vi "TEST_cRIO.vi"() -> ()   [LabVIEW 2017]
uses:
  <vilib>/Analysis/baseanly.llb/Mean (DBL).vi
  <vilib>/Analysis/NI_AALBase.lvlib
panel:
  in  "Boolean":bool
  out "R3(kOhm)":dbl format="%.1f"
  out "R2(kOhm)":dbl format="%.1f"
  out "R1(kOhm)":dbl format="%.1f"
  out "Corriente(mA)":dbl format="%.3f"
  in  "AO0":dbl format="%.2f"
  out "AI3(V)":dbl format="%.6f"
  out "AI2(V)":dbl format="%.6f"
  out "AI1(V)":dbl format="%.6f"
  out "Waveform Chart":cluster{dbl, dbl, dbl}(graph)
  in  "Period":dbl=0.1 format="%.1f"
  in  "stop":bool
  out "AI0(V)":dbl format="%.6f"
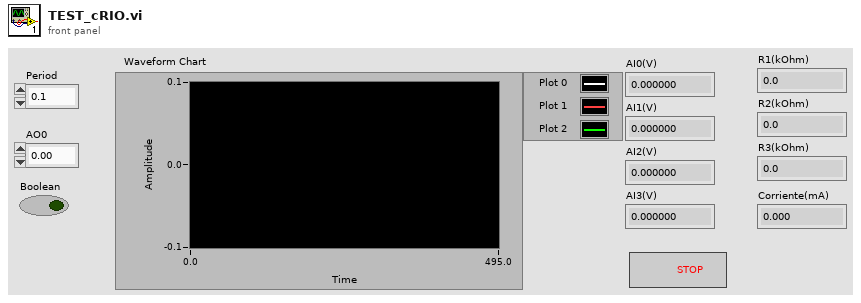
[diagram p1: front panel]
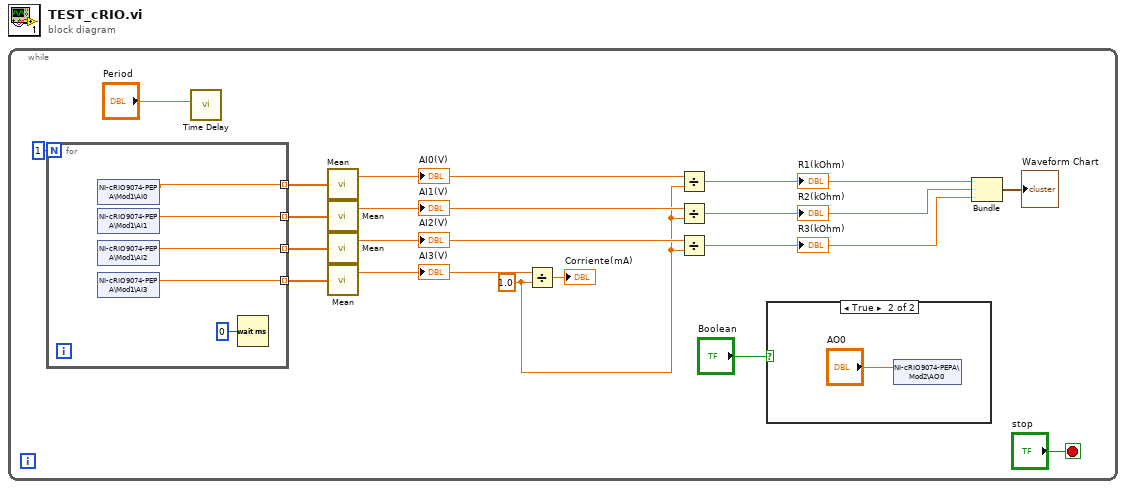
[diagram p0: block diagram]
diagram:
  n1 = while {
    stop <- "stop" stop-if-true
    w3 = 1.0 ("y")
    n2 = for {
      N: 1 -> [_]
      tunnel: [w20] -> w14 mode=indexing
      tunnel: [w21] -> w12 mode=indexing
      tunnel: [w22] -> w11 mode=indexing
      tunnel: [w23] -> w10 mode=indexing
      n3 = shared-variable "NI-cRIO9074-PEPA\\Mod1\\AI0"() -> (w20:dbl)  [unwired: 1 in, 1 out]
      n4 = shared-variable "NI-cRIO9074-PEPA\\Mod1\\AI1"() -> (w21:dbl)  [unwired: 1 in, 1 out]
      n5 = shared-variable "NI-cRIO9074-PEPA\\Mod1\\AI2"() -> (w22:dbl)  [unwired: 1 in, 1 out]
      n6 = shared-variable "NI-cRIO9074-PEPA\\Mod1\\AI3"() -> (w23:dbl)  [unwired: 1 in, 1 out]
      n7 = Wait (ms)(milliseconds to wait=u32 0) -> ()  [unwired: 1 out]
    }
    n8 = call "Time Delay"("Delay Time (s)"="Period") -> ()  [unwired: 10 in, 1 out]
    n9 = call-poly <vilib>:"Mean.vi"("X"=w14) -> ("mean"=w13:dbl)  [unwired: 1 out]
    "AI0(V)" <- w13
    n10 = call-poly <vilib>:"Mean.vi"("X"=w12) -> ("mean"=w8:dbl)  [unwired: 1 out]
    "AI1(V)" <- w8
    n11 = call-poly <vilib>:"Mean.vi"("X"=w11) -> ("mean"=w7:dbl)  [unwired: 1 out]
    "AI2(V)" <- w7
    n12 = call-poly <vilib>:"Mean.vi"("X"=w10) -> ("mean"=w9:dbl)  [unwired: 1 out]
    "AI3(V)" <- w9
    n13 = Divide(x=w9, y=w3) -> (x/y=→"Corriente(mA)":dbl)
    n14 = Divide(x=w13, y=w3) -> (x/y=w6:dbl)
    "R1(kOhm)" <- w6
    n15 = Divide(x=w8, y=w3) -> (x/y=w5:dbl)
    "R2(kOhm)" <- w5
    n16 = Divide(x=w7, y=w3) -> (x/y=w4:dbl)
    "R3(kOhm)" <- w4
    n17 = case shown="True" "Boolean" {
      frame False {
      }
      frame True {
        n18 = shared-variable "NI-cRIO9074-PEPA\\Mod2\\AO0"("AO0") -> ()  [unwired: 1 in, 1 out]
      }
    }
    n19 = Bundle(w6, w5, w4) -> (→"Waveform Chart":cluster{dbl, dbl, dbl})  [unwired: 1 in]
  }
